vi "Recurse.vi"(6 "Teller":refnum<class "Teller.lvclass">, 7 "Actor in":refnum<class "Actor.lvclass">, 8 "Error in":errorcluster) -> (0 "Error out":errorcluster, 5 "Actor out":refnum<class "Actor.lvclass">)   [LabVIEW 2020, in "_Template.lvlib" / "Templates.lvlib" / "TEMPLATE jettl Msg.lvlib" / "TEMPLATE.lvlib"]
uses:
  TEMPLATE.lvlib
  jettl/jettl/Actor/Actor.lvclass
  jettl/jettl/Teller/Teller.lvclass
  jettl/jettl/jettl.lvlib
  TEMPLATE Msg Output/TEMPLATE Msg Output.lvlib
  Init Msg.vi
panel:
  # "This front panel should not be manipulated."
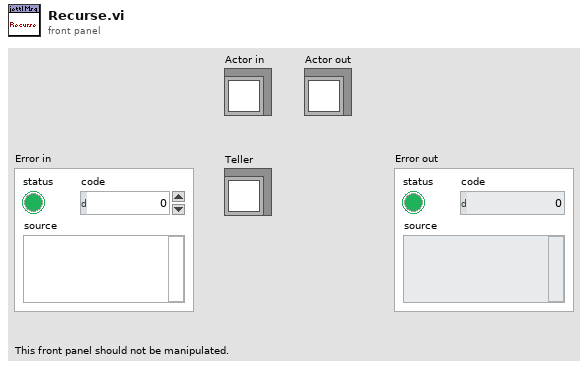
[diagram p1: front panel]
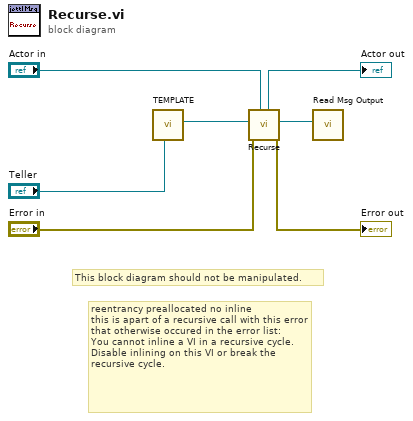
[diagram p0: block diagram]
diagram:
  # "This block diagram should not be manipulated."
  # "reentrancy preallocated no inline\nthis is apart of a recursive call with this error that otherwise occured in the error list:\nYou cannot inline a VI in a recursive cycle. Disable inlining on this VI or break the recursive cycle."
  n1 = call-poly "TEMPLATE.vi"("Teller"="Teller") -> ("Msg"=w3:refnum<class "Msg.lvclass">)  [unwired: 10 in]
  n2 = call "Recurse.vi"("Actor in"="Actor in", "Error in"="Error in", "Msg"=w3) -> ("Error out"=→"Error out":errorcluster, "Msg Output"=w4:refnum<class "Msg Output.lvclass">, "Actor out"=→"Actor out":refnum<class "Actor.lvclass">)  [unwired: 6 in]
  n3 = call "Read Msg Output.vi"("Msg Output"=w4) -> ()  [unwired: 11 in]
